vi "SHA-224.vi"() -> (0 "Hash Function out":refnum<class "NI_SHA-256.lvclass">)   [LabVIEW 2013, in "NI_SHA-256(2013).lvlib" / "NI_SHA-256.lvclass"]
doc: "Returns an instance of the SHA-224 hash function."
uses:
  NI_SHA-256.lvclass
  subVIs/Mode.ctl
  NI_SHA-256.lvclass/NI_SHA-256.ctl
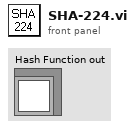
[diagram p1: front panel]
types:
  T1 = typedef "NI_SHA-256(2013).lvlib/NI_SHA-256.lvclass/Mode.ctl" = enum16{"SHA-256", "SHA-224"}
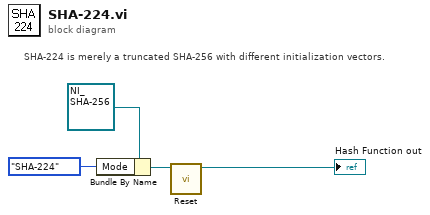
[diagram p0: block diagram]
diagram:
  # "SHA-224 is merely a truncated SHA-256 with different initialization vectors."
  n1 = Bundle By Name(cluster=refnum<class "NI_SHA-256.lvclass"> refnum ("nihash-sha2.lvlib:SHA-256.lvclass"), "Mode"=Mode."SHA-224") -> (w2:refnum<class "NI_SHA-256.lvclass">)
  n2 = call "Reset.vi"("Hash Function in"=w2) -> ("Hash Function out"=→"Hash Function out":refnum<class "NI_SHA-256.lvclass">)  [unwired: 10 in]
